vi "CS++Main.vi"() -> ()   [LabVIEW 2016]
doc: "This VI illustrates how to use the <b>Launch CS++StartActor.vi</b> as subVI.\n\nYou may create a copy and add your project specific stuff."
uses:
  Packages/CSPP_Core/Libraries/Base/Severity.ctl
  Packages/CSPP_Core/Actors/CS++StartActor/CS++StartActor.lvlib
  Packages/CSPP_Core/Libraries/Base/CS++Base.lvlib
panel:
  in  "Debug Level":T1=enum."warning"
  out "Attributes found?":bool
  out "Error Out":errorcluster
  in  "Error In":errorcluster
  in  "CS++Factory":path
  in  "Start Actor":string="CS++StartActor"
  in  "DB Connection String":string
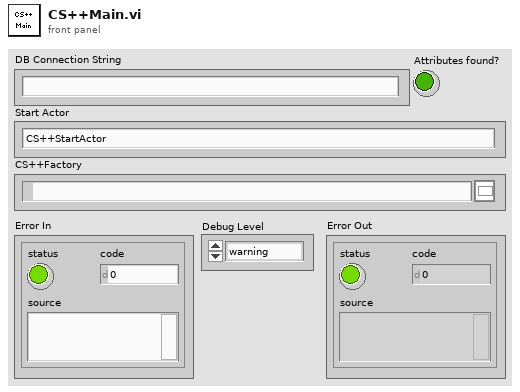
[diagram p1: front panel]
types:
  T1 = typedef "CS++Base.lvlib/Severity.ctl" = enum16{"emergency", "alert", "critical", "error", "warning", "notice", "info", "debug"}
  T2 = cluster{"Classname":string, "CS++Messages":refnum<class "Message.lvclass">[]}[]
  T3 = enum32{"invalid app kind", "Development System", "Run Time System", "Student Edition", "Embedded LabVIEW", "Evaluation", "Custom"}
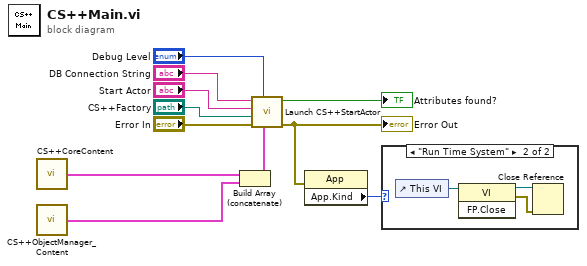
[diagram p0: block diagram]
diagram:
  n1 = call "CS++CoreContent.vi"() -> ("CS++Classes & Messages"=w4:T2)  [unwired: 1 in]
  n2 = call "CS++ObjectManager_Content.vi"() -> ("CS++Classes & Messages"=w6:T2)  [unwired: 1 in]
  n3 = Build Array (concatenate)(w4, w6) -> (w5:T2)
  n4 = call "Launch CS++StartActor.vi"("CS++Classes & Messages"=w5, "Debug Level"="Debug Level", "Error In"="Error In", "CS++Factory"="CS++Factory", "Start Actor"="Start Actor", "DB Connection String"="DB Connection String") -> ("Error Out"=w1:errorcluster, "Attributes found?"=→"Attributes found?":bool)  [unwired: 3 in, 1 out]
  "Error Out" <- w1
  n5 = property class="App"(error in=w1) -> ("App.Kind"=w2:T3)  [unwired: 1 in, 2 out]
  n6 = case shown="\"Run Time System\"" w2 {
    frame Default {
    }
    frame "Run Time System" {
      n7 = control-ref of="This VI"() -> (w14:refnum<vi>)
      n8 = invoke class="VI" method="FP.Close"(reference=w14) -> (reference out=w13:refnum<vi>, error out=w12:errorcluster)  [unwired: 2 in, 1 out]
      n9 = Close Reference(reference=w13, error in (no error)=w12) -> ()  [unwired: 1 out]
    }
  }
